vi "Tokenization.vi"(8 "error in (no error)":errorcluster, 11 "string":string) -> (0 "error out":errorcluster, 3 "tokens":string[](array[string]))   [LabVIEW 2017]
uses:
  <vilib>/regexp/Match Regular Expression.xnode
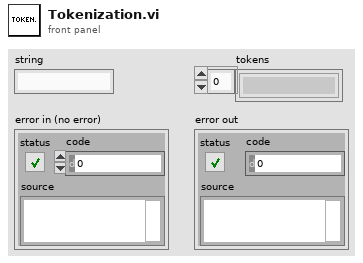
[diagram p1: front panel]
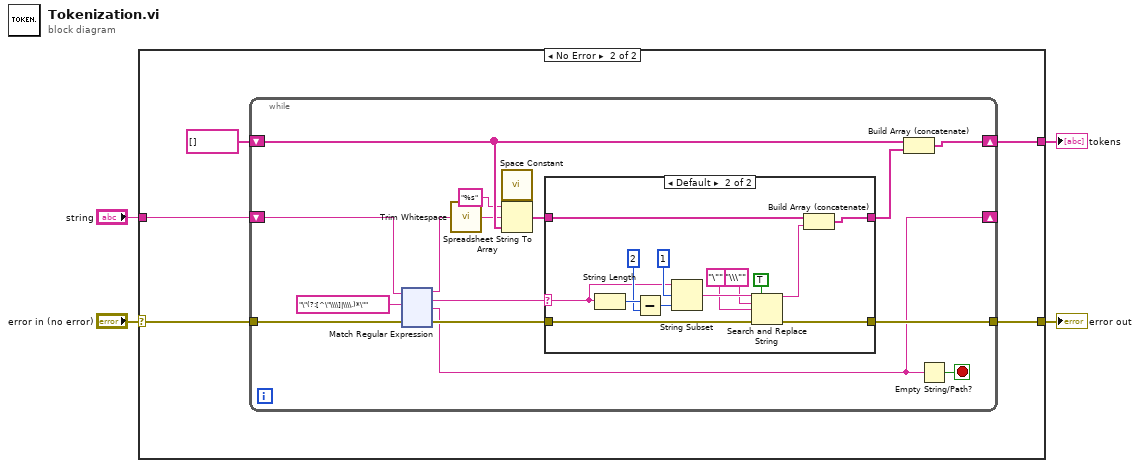
[diagram p0: block diagram]
diagram:
  n1 = case shown="No Error" "error in (no error)" {
    selector: "error in (no error)" -> [w5 w6]
    tunnel: "string" -> [_ w10]
    tunnel: [_ w8] -> w3
    tunnel: [w5 w7] -> w1
    frame Error {
    }
    frame No Error {
      n2 = while {
        shift-right: [w22] -> _
        shift-left: w10 -> [w13]
        shift-right: [w20] -> w8
        shift-left: string[] [] -> [w24]
        tunnel: [w25] -> w7
        tunnel: w6 -> [w11]
        stop <- w21 stop-if-true
        n3 = xnode "Match Regular Expression"("input string"=w13, "regular expression"="\"(?:[^\"\\\\]|\\\\.)*\"", "error in"=w11) -> ("before match"=w12:string, "whole match"=w19:string, "after match"=w22:string, "error out"=w26:errorcluster)  [unwired: 3 in, 1 out]
        n4 = call <vilib>:"Trim Whitespace.vi"("string"=w12) -> ("trimmed string"=w14:string)  [unwired: 1 in]
        n5 = call <vilib>:"Space Constant.vi"() -> ("String"=w15:string)
        n6 = Spreadsheet String To Array(delimiter (Tab)=w15, format string="%s", spreadsheet string=w14, array type (2D Dbl)=w24) -> (array=w16:string[])
        n7 = case shown="Default" w19 {
          selector: w19 -> [_ w29]
          tunnel: w16 -> [w28 w34]
          tunnel: [w28 w32] -> w18
          tunnel: w26 -> [w27 w31]
          tunnel: [w27 w30] -> w25
          frame "" {
          }
          frame Default {
            n8 = String Length(string=w29) -> (length=w41:i32)
            n9 = Subtract(x=w41, y=2 ("x")) -> (x-y=w40:i32)
            n10 = String Subset(string=w29, offset (0)=1, length (rest)=w40) -> (substring=w38:string)
            n11 = Search and Replace String(replace all?=TRUE ("replace all? (F)"), input string=w38, search string="\\\"", replace string="\"" ("replace string (\"\")"), error in=w31) -> (result string=w33:string, error out=w30:errorcluster)  [unwired: 3 in, 2 out]
            n12 = Build Array (concatenate)(w34, w33) -> (w32:string[])
          }
        }
        n13 = Build Array (concatenate)(w24, w18) -> (w20:string[])
        n14 = Empty String/Path?(string/path=w22) -> (empty?=w21:bool)
      }
    }
  }
  "tokens" <- w3
  "error out" <- w1
